vi "Terminate State Machine.vi"(8 "error in (no error)":errorcluster, 10 "Loaded Plugins In":refnum<class "Generic Plugin.lvclass">[](array[class]), 11 "User Interface References":T1) -> (0 "error out":errorcluster, 3 "User Interface References Out":T1)   [LabVIEW 2011]
uses:
  <vilib>/Utility/config.llb/NI_LVConfig.lvlib
  Sliding Menu Type Definitions/User Interface Type Definitions.ctl
  <vilib>/Utility/config.llb/Config Data RefNum.ctl
  Parent Plugin Definition/Plugin Template/Generic Plugin.lvclass
  Button XControl.xctl
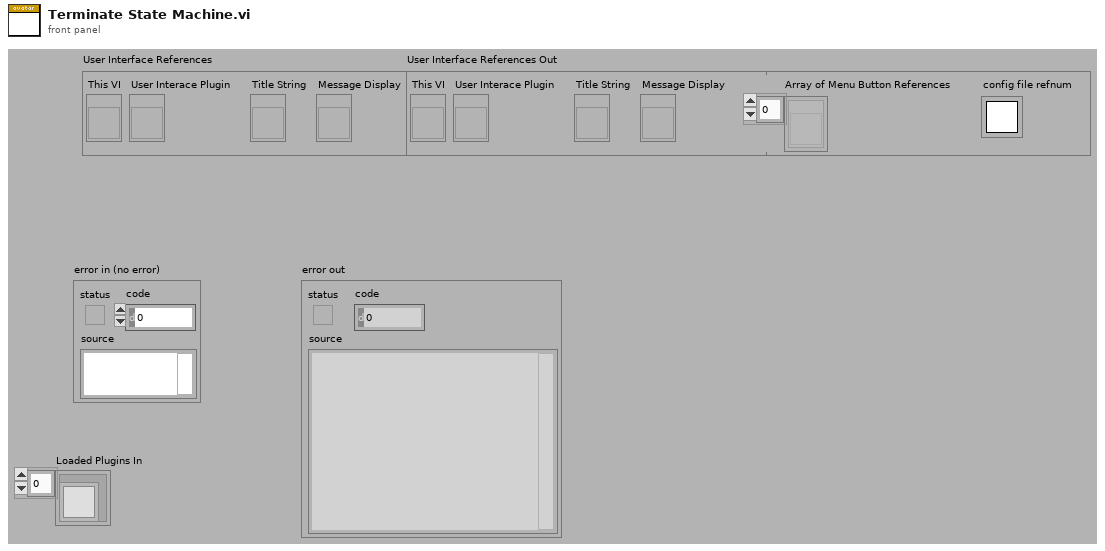
[diagram p1: front panel]
types:
  T1 = typedef "Sliding Menu Project Library.lvlib/User Interface Type Definitions.ctl" = cluster{"This VI":refnum<vi>, "User Interace Plugin":refnum<vi>, "Title String":refnum<vi>, "Message Display":refnum<vi>, "Array of Menu Button References":refnum<vi>[], "config file refnum":T2}
  T2 = typedef "NI_LVConfig.lvlib/Config Data RefNum.ctl" = refnum<k1>
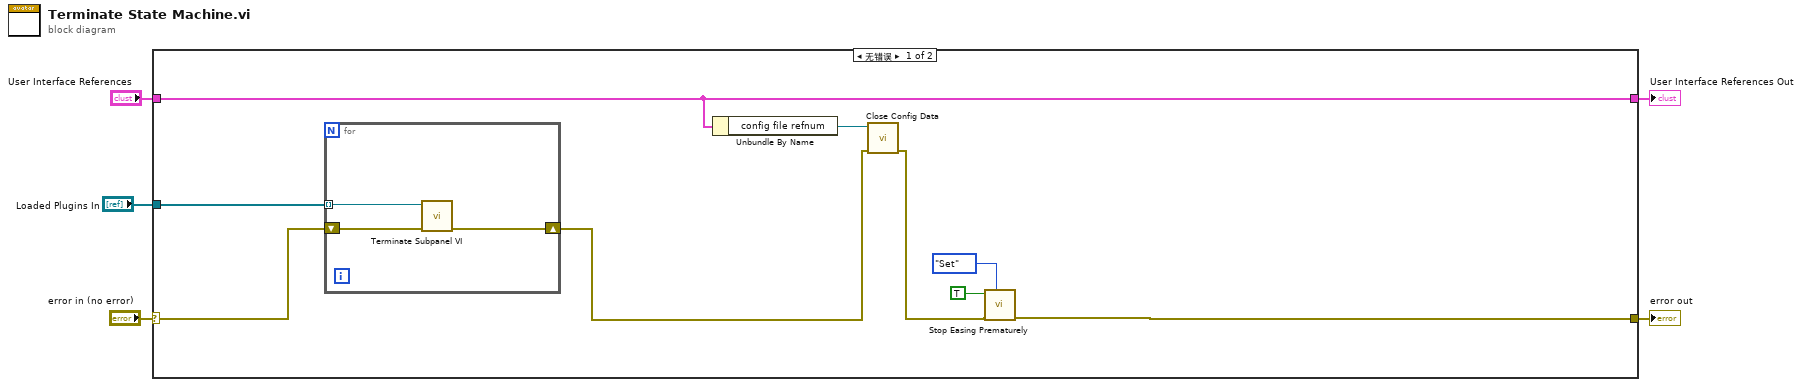
[diagram p0: block diagram]
diagram:
  n1 = case shown="无错误" "error in (no error)" {
    selector: "error in (no error)" -> [w8 w19]
    tunnel: [w6 w19] -> w5
    tunnel: [w10 w18] -> w2
    tunnel: "User Interface References" -> [w10 w18]
    tunnel: "Loaded Plugins In" -> [w9 _]
    frame No Error {
      n2 = for {
        tunnel: w9 -> [w17] mode=indexing
        shift-right: [w15] -> w7
        shift-left: w8 -> [w16]
        n3 = call "Terminate Subpanel VI.vi"("error in (no error)"=w16, "Generic Plugin in"=w17) -> ("error out"=w15:errorcluster)  [unwired: 8 in, 1 out]
      }
      n4 = Unbundle By Name(w10) -> ("config file refnum"=w14:T2)
      n5 = call <vilib>:"Close Config Data.vi"("error in (no error)"=w7, "refnum"=w14) -> ("error out"=w11:errorcluster)  [unwired: 8 in, 1 out]
      n6 = call "Stop Easing Prematurely.vi"("Set or Get Value"=enum16{"Set", "Get"}."Set", "error in"=w11, "Stop?"=TRUE) -> ("error out"=w6:errorcluster)  [unwired: 7 in, 1 out]
    }
    frame Error {
    }
  }
  "error out" <- w5
  "User Interface References Out" <- w2
